vi "mediano.vi"(11 "data":dbl[](array[numeric]) format="%.10f") -> (1 "Q3":dbl format="%.10f", 2 "median":dbl format="%.10f", 3 "Q1":dbl format="%.10f")   [LabVIEW 2021, in "statistics.lvlib"]
uses:
  statistics.lvlib
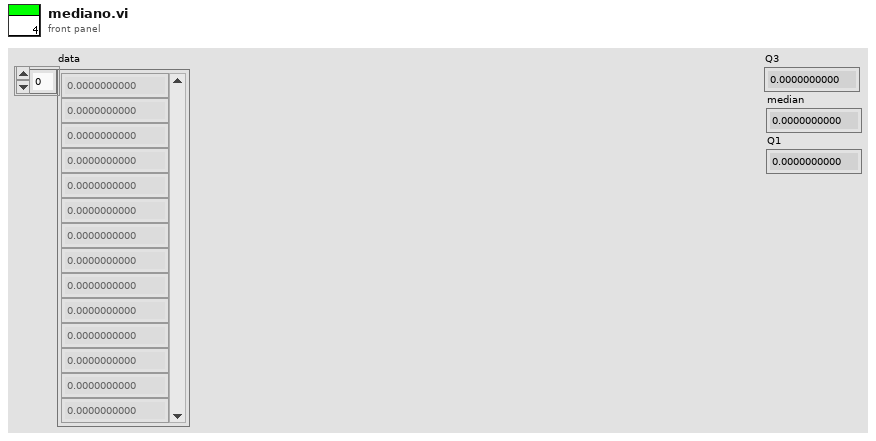
[diagram p1: front panel]
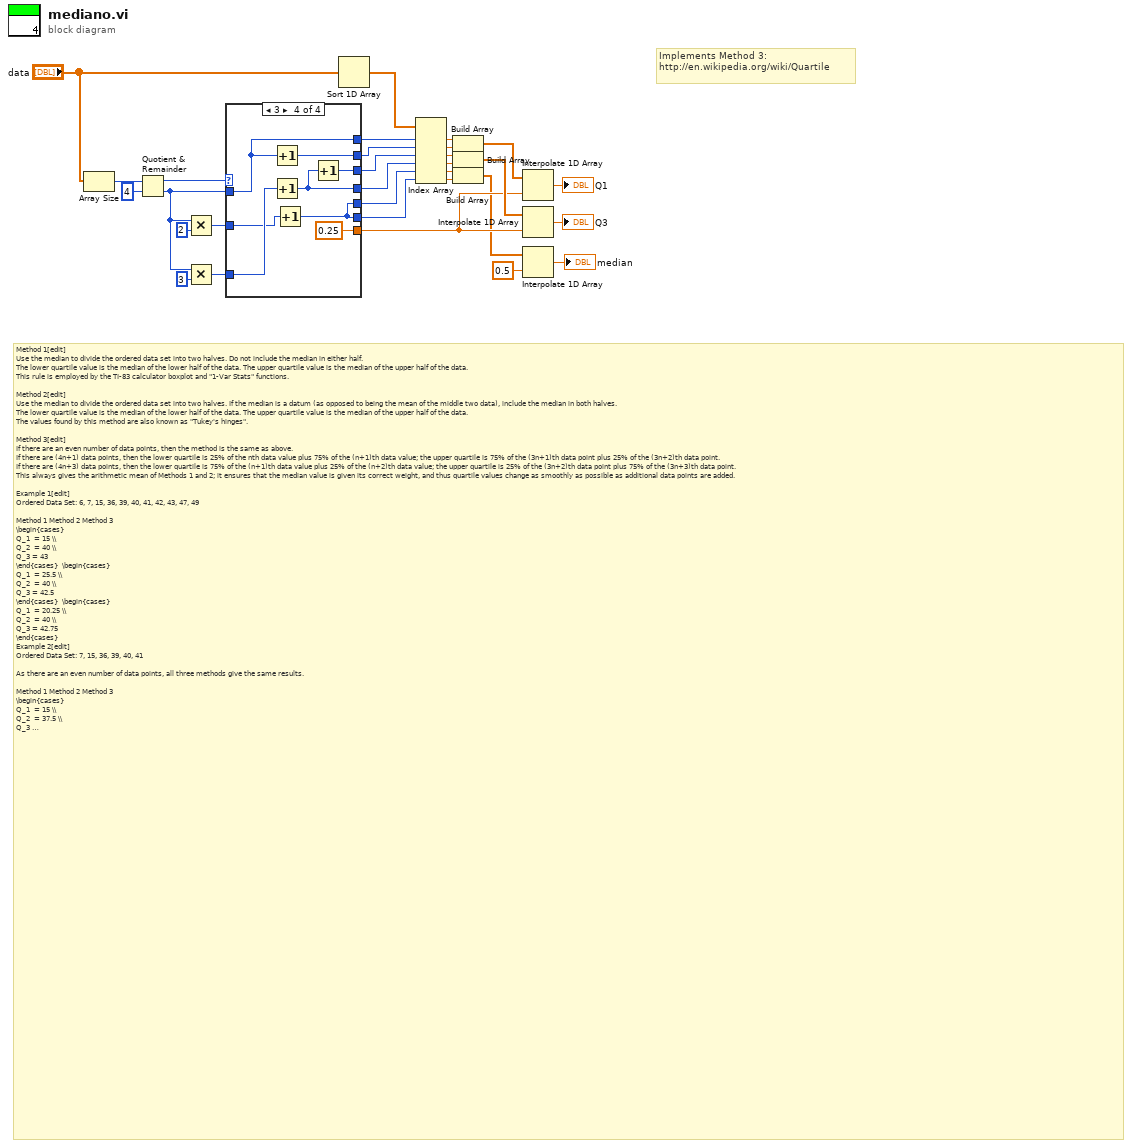
[diagram p0: block diagram]
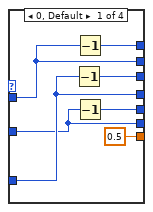
[diagram p2: hidden frame]
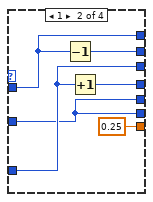
[diagram p3: hidden frame]
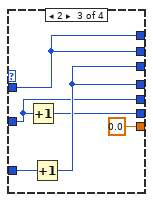
[diagram p4: hidden frame]
diagram:
  # "Method 1[edit]\nUse the median to divide the ordered data set into two halves. Do not include the median in either half.\nThe lower quartile value is the median of the lower half of the data. The upper quartile value is the median of the upper half of the data.\nThis rule is employed by the TI-83 calculator boxplot and \"1-Var Stats\" functions.\n\nMethod 2[edit]\nUse the median to divide the ordered data set into two halves. If the median is a datum (as opposed to being the mean of the middle two data), include the median in both halves.\nThe lower quartile value is the median of the lower half of the data. The upper quartile value is the median of the upper half of the data.\nThe values found by this method are also known as \"Tukey's hinges\".\n\nMethod 3[edit]\nIf there are an even number of data points, then the method is the same as above.\nIf there are (4n+1) data points, then the lower quartile is 25% of the nth data value plus 75% of the (n+1)th data value; the upper quartile is 75% of the (3n+1)th data point plus 25% of the (3n+2)th data point.\nIf there are (4n+3) data points, then the lower quartile is 75% of the (n+1)th data value plus 25% of the (n+2)th data value; the upper quartile is 25% of the (3n+2)th data point plus 75% of the (3n+3)th data point.\nThis always gives the arithmetic mean of Methods 1 and 2; it ensures that the median value is given its correct weight, and thus quartile values change as smoothly as possible as additional data points are added.\n\nExample 1[edit]\nOrdered Data Set: 6, 7, 15, 36, 39, 40, 41, 42, 43, 47, 49\n\nMethod 1\tMethod 2\tMethod 3\n\\begin{cases}\nQ_1  = 15 \\\\\nQ_2  = 40 \\\\\nQ_3 = 43\n\\end{cases} \t\\begin{cases}\nQ_1  = 25.5 \\\\\nQ_2  = 40 \\\\\nQ_3 = 42.5\n\\end{cases} \t\\begin{cases}\nQ_1  = 20.25 \\\\\nQ_2  = 40 \\\\\nQ_3 = 42.75\n\\end{cases} \nExample 2[edit]\nOrdered Data Set: 7, 15, 36, 39, 40, 41\n\nAs there are an even number of data points, all three methods give the same results.\n\nMethod 1\tMethod 2\tMethod 3\n\\begin{cases}\nQ_1  = 15 \\\\\nQ_2  = 37.5 \\\\\nQ_3 = 40\n\\end{cases} \t\\begin{cases}\nQ_1 = 15 \\\\\nQ_2 = 37.5 \\\\\nQ_3 = 40\n\\end{cases} \t\\begin{cases}\nQ_1 = 15.0 \\\\\nQ_2 = 37.5 \\\\\nQ_3 = 40.0\n\\end{cases}"
  # "Implements Method 3:\nhttp://en.wikipedia.org/wiki/Quartile"
  n1 = Array Size(array="data") -> (size(s)=w29:i32)
  n2 = Quotient & Remainder(x=w29, y=4) -> (x-y*floor(x/y)=w27:i32, floor(x/y)=w6:i32)
  n3 = Multiply(x=w6, y=2) -> (x*y=w5:i32)
  n4 = Multiply(x=w6, y=3) -> (x*y=w14:i32)
  n5 = case shown="3" w27 {
    tunnel: w6 -> [w37 w42 w49 w56]
    tunnel: [w35 w42 w49 w56] -> w19
    tunnel: [w37 w39 w49 w57] -> w18
    tunnel: [w33 w41 w46 w54] -> w17
    tunnel: [w36 w40 w46 w52] -> w16
    tunnel: w14 -> [w36 w41 w48 w53]
    tunnel: [0.5 0.25 0.0 0.25] -> w13
    tunnel: w5 -> [w31 w38 w45 w51]
    tunnel: [w32 w38 w45 w50] -> w3
    tunnel: [w31 w38 w44 w50] -> w2
    frame 0, Default {
      n6 = Decrement(x=w36) -> (x-1=w33:i32)
      n7 = Decrement(x=w37) -> (x-1=w35:i32)
      n8 = Decrement(x=w31) -> (x-1=w32:i32)
    }
    frame 1 {
      n9 = Decrement(x=w42) -> (x-1=w39:i32)
      n10 = Increment(x=w41) -> (x+1=w40:i32)
    }
    frame 2 {
      n11 = Increment(x=w45) -> (x+1=w44:i32)
      n12 = Increment(x=w48) -> (x+1=w46:i32)
    }
    frame 3 {
      n13 = Increment(x=w56) -> (x+1=w57:i32)
      n14 = Increment(x=w53) -> (x+1=w52:i32)
      n15 = Increment(x=w51) -> (x+1=w50:i32)
      n16 = Increment(x=w52) -> (x+1=w54:i32)
    }
  }
  n17 = Sort 1D Array(array="data") -> (sorted array=w26:dbl[])
  n18 = Index Array(array=w26, index #1=w19, index #2=w18, index #3=w17, index #4=w16, index #5=w3, index #6=w2) -> (element #1=w25:dbl, element #2=w24:dbl, element #3=w23:dbl, element #4=w22:dbl, element #5=w10:dbl, element #6=w9:dbl)
  n19 = Build Array(w25, w24) -> (w21:dbl[])
  n20 = Build Array(w23, w22) -> (w20:dbl[])
  n21 = Build Array(w10, w9) -> (w8:dbl[])
  n22 = Interpolate 1D Array(1:w13, 2:w21) -> (0:→"Q1":dbl)
  n23 = Interpolate 1D Array(1:w13, 2:w20) -> (0:→"Q3":dbl)
  n24 = Interpolate 1D Array(1:0.5 ("fractional index or x"), 2:w8) -> (0:→"median":dbl)
